vi "initialize Session Data.vi"(0 "Session in":refnum<class "Engine.lvclass">, 11 "error in":errorcluster) -> (4 "Session out":refnum<class "Engine.lvclass">, 15 "error out":errorcluster)   [LabVIEW 2020, in "HTS.lvlib" / "Engine.lvclass"]
uses:
  Engine.lvclass
  <userlib>/_Session Fwk/Session - Root.lvclass
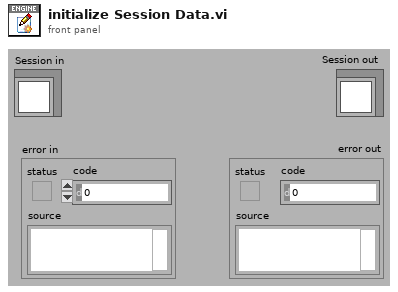
[diagram p1: front panel]
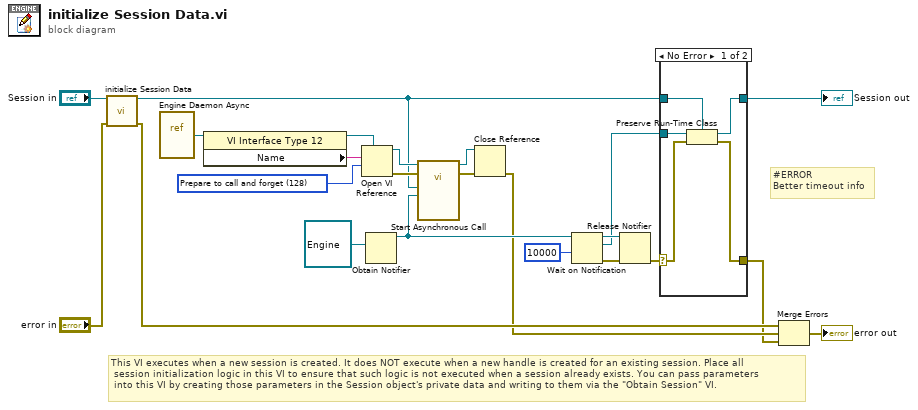
[diagram p0: block diagram]
diagram:
  w15 = 128 items=["Record modifications"=1, "Open templates for editing"=2, "Prompt user to save"=4, "Prepare for reentrant run"=8, "Prompt to find missing subVIs"=16, "Hide loading dialog box"=32, "Enable simultaneous calls"=64, "Prepare to call and forget"=128, "Simultaneous call and forget"=192, "Prepare to call and collect"=256, "Simultaneous call and collect"=320]
  # "#ERROR\nBetter timeout info"
  # "This VI executes when a new session is created. It does NOT execute when a new handle is created for an existing session. Place all\n session initialization logic in this VI to ensure that such logic is not executed when a session already exists. You can pass parameters\n into this VI by creating those parameters in the Session object's private data and writing to them via the \"Obtain Session\" VI."
  n1 = call-parent "initialize Session Data.vi"("OBJ - Session in"="Session in", "error in"="error in") -> ("OBJ - Session out"=w1:refnum<class "Engine.lvclass">, "error out"=w23:errorcluster)  [unwired: 12 in]
  n2 = vi-ref "Engine Daemon Async.vi"() -> (w13:refnum<vi>)
  n3 = property class="VI Interface Type 12"(reference=w13) -> (reference out=w16:refnum<vi>, "Name"=w14:string)  [unwired: 1 in, 1 out]
  n4 = Open VI Reference(type specifier VI Refnum (for type only)=w16, vi path=w14, options=w15) -> (vi reference=w18:refnum<vi>, error out=w17:errorcluster)  [unwired: 3 in]
  n5 = Obtain Notifier(notification data type=refnum<class "Engine.lvclass"> refnum ("TSEngine")) -> (notifier out=w7:refnum<notifier>)  [unwired: 3 in, 2 out]
  n6 = call-by-ref "Start Asynchronous Call"(reference=w18, error in=w17, "Daemon Notifier"=w7, "TSEngine in"=w1) -> (reference out=w20:refnum<vi>, error out=w19:errorcluster)  [unwired: 10 in]
  n7 = Close Reference(reference=w20, error in (no error)=w19) -> (error out=w6:errorcluster)
  n8 = Wait on Notification(notifier=w7, timeout in ms (-1)=10000) -> (notifier out=w12:refnum<notifier>, notification=w4:refnum<class "Engine.lvclass">, error out=w11:errorcluster)  [unwired: 2 in, 1 out]
  n9 = Release Notifier(notifier=w12, error in (no error)=w11) -> (error out=w5:errorcluster)  [unwired: 1 in, 2 out]
  n10 = case shown="No Error" w5 {
    selector: w5 -> [w25 w29]
    tunnel: w4 -> [w28 _]
    tunnel: w1 -> [w27 w30]
    tunnel: [w26 w30] -> w3
    tunnel: [w24 w29] -> w2
    frame No Error {
      n11 = Preserve Run-Time Class(object in=w28, error in=w25, 2:w27) -> (object out=w26:refnum<class "Engine.lvclass">, error out=w24:errorcluster)
    }
    frame Error {
    }
  }
  "Session out" <- w3
  n12 = Merge Errors(w23, w6, w2) -> (→"error out":errorcluster)
